vi "Downsample_Filter_Test.vi"() -> ()   [LabVIEW 2018]
uses:
  <vilib>/measure/maspectr.llb/Power Spectrum and PSD Export Mode.ctl
  <vilib>/measure/maspectr.llb/FFT Power Spectrum and PSD for 1 Chan.vi
  <vilib>/measure/NI_MAPro.lvlib
panel:
  out "original size":i32
  out "filtered size":i32
  out "Output valid":i16[](graph)
  out "filtered numeric":dbl[](array[numeric])
  out "Filtered signal":dbl[](graph)
  out "Power spectrum in":cluster{"f0":dbl, "df":dbl, "magnitude":dbl[]}(graph)
  out "Power spectrum out":cluster{"f0":dbl, "df":dbl, "magnitude":dbl[]}[](graph)
  out "Input signal":dbl[](graph)
  out "# of Iterations":i32
  out "# of samples":i32
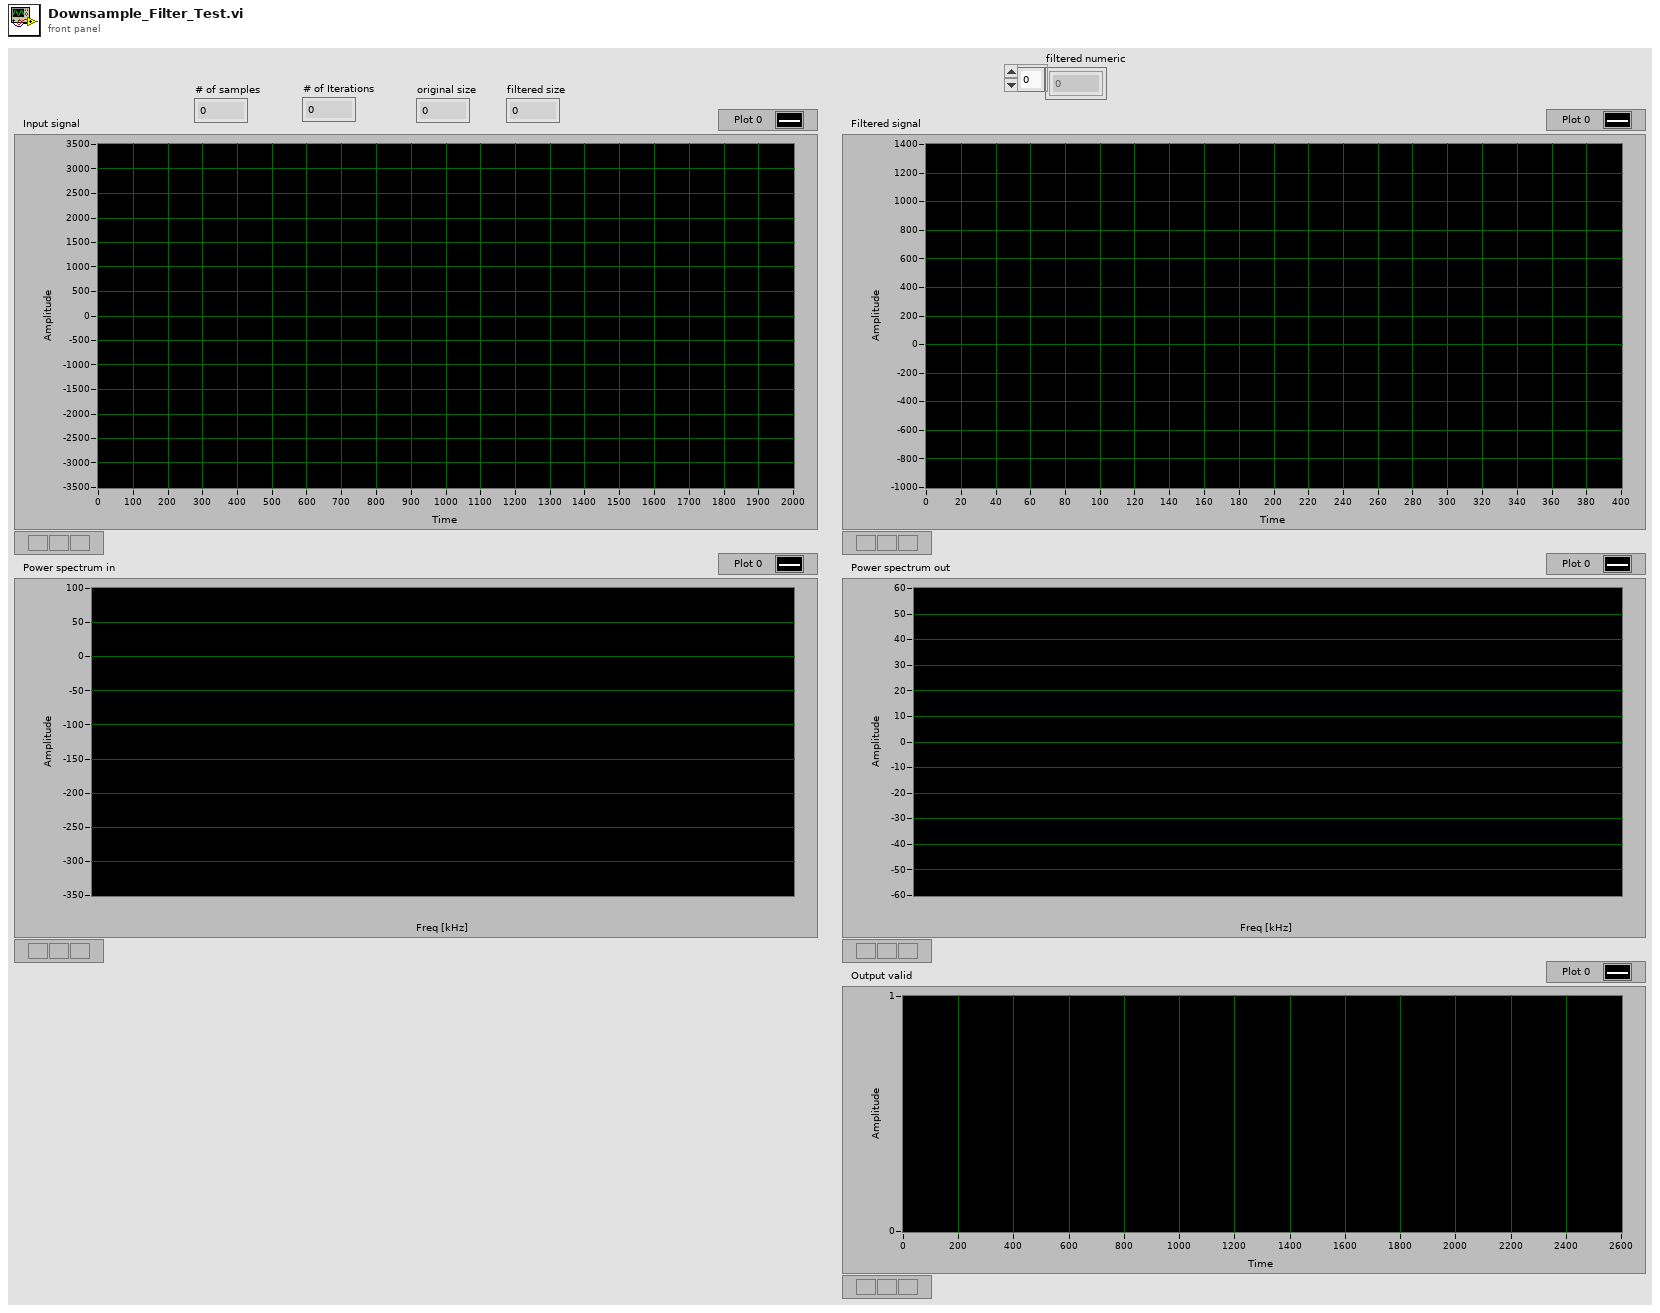
[diagram p1: front panel]
types:
  T1 = typedef "NI_MAPro.lvlib/Power Spectrum and PSD Export Mode.ctl" = u16
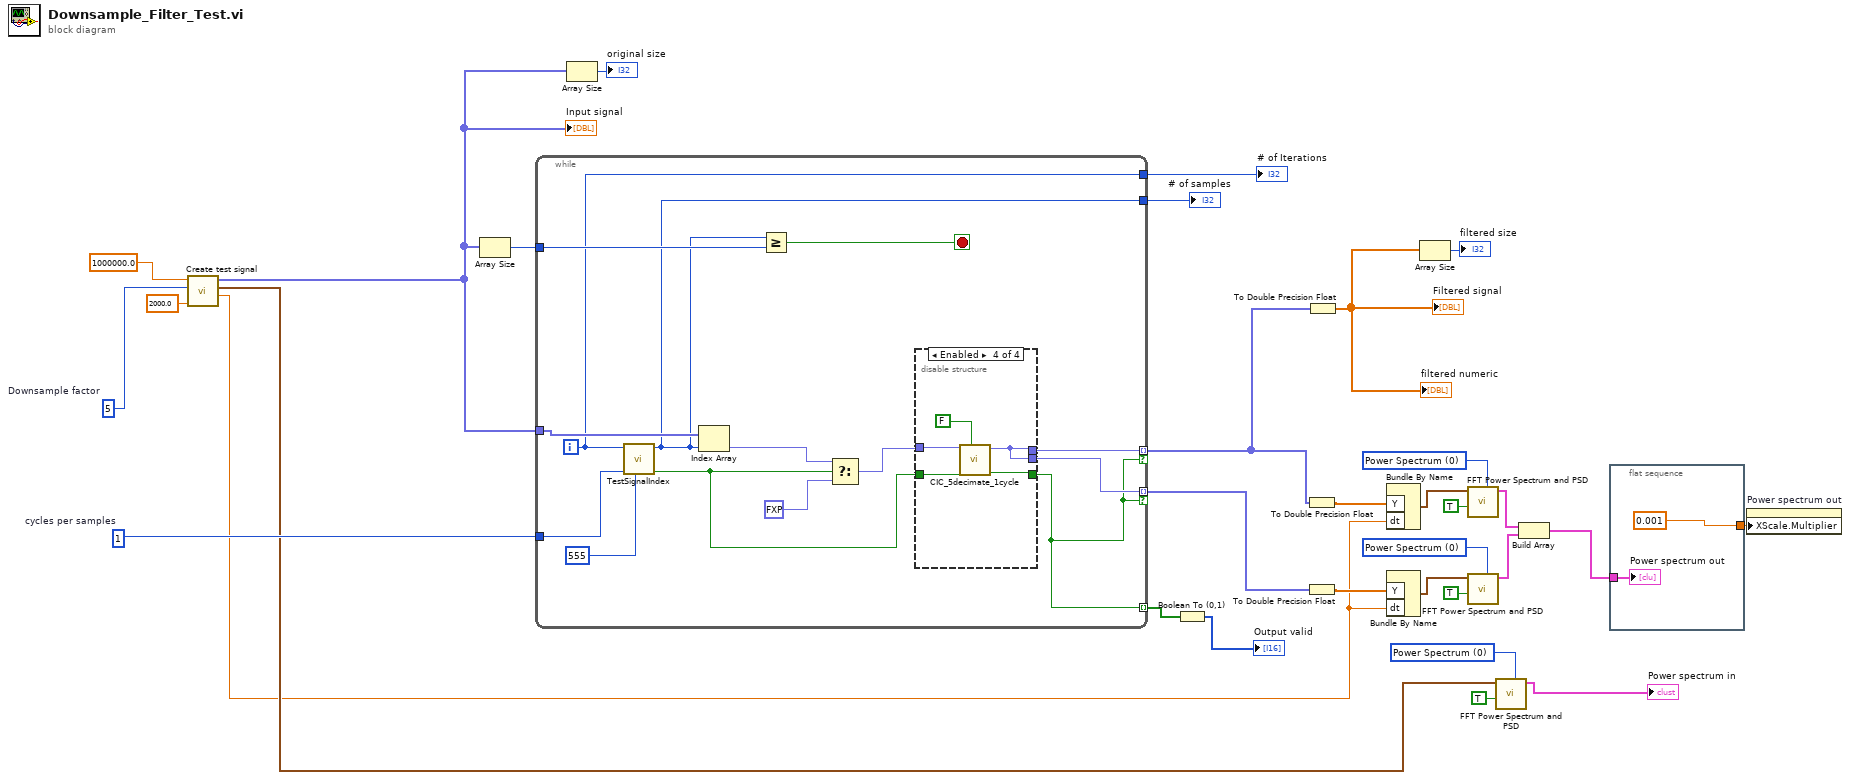
[diagram p0: block diagram]
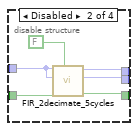
[diagram p3: hidden frame]
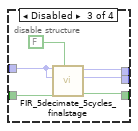
[diagram p4: hidden frame]
diagram:
  w15 = T1 0 items=["Power Spectrum", "Power Spectral Density"] ("export mode")
  w20 = 5  # Downsample factor
  w24 = 1  # cycles per samples
  w26 = T1 0 items=["Power Spectrum", "Power Spectral Density"] ("export mode")
  w30 = T1 0 items=["Power Spectrum", "Power Spectral Density"] ("export mode")
  n1 = call "Create test signal.vi"("Number of samples"=2000.0, "Downsample factor"=w20, "Sample rate"=1000000.0) -> ("dt"=w9:dbl, "signal out"=w22:waveform(dbl), "Y"=w4:fxp<+/-,16,14>[])  [unwired: 6 in]
  "Input signal" <- w4
  n2 = Array Size(array=w4) -> (size(s)=w32:i32)
  n3 = while {
    tunnel: w4 -> [w46]
    tunnel: [w43] -> w12 mode=indexing if=w35
    tunnel: w32 -> [w44]
    tunnel: w24 -> [w42]
    tunnel: [w35] -> w23 mode=indexing
    tunnel: [w36] -> w11 mode=indexing if=w35
    tunnel: [w34] -> w3
    tunnel: [w33] -> w2
    i -> [w33]
    stop <- w45 stop-if-true
    n4 = call "TestSignalIndex.vi"("initial delay"=555, "cycles per sample"=w42, "index"=w33) -> ("valid out"=w37:bool, "array index"=w34:i32)  [unwired: 7 in]
    n5 = Index Array(array=w46, index=w34) -> (element=w41:fxp<+/-,16,14>)
    n6 = Greater Or Equal?(x=w34, y=w44) -> (x >= y?=w45:bool)
    n7 = Select(t=w41, s=w37, f=fxp<+/-,16,14> 0.0) -> (s? t:f=w40:fxp<+/-,16,14>)
    n8 = disable-structure shown="Enabled" {
      disable-tunnel: [w51 w56 w62 w66] -> w43
      disable-tunnel: w40 -> [w50 w55 w61 w70]
      disable-tunnel: w37 -> [w49 w58 w64 w68]
      disable-tunnel: [w48 w54 w60 w66] -> w36
      disable-tunnel: [w47 w57 w63 w67] -> w35
      frame Disabled {
        n9 = flat-sequence {
          tunnel: [w53] -> w51
          tunnel: w50 -> [w53]
          tunnel: w49 -> [w52]
          tunnel: [w53] -> w48
          tunnel: [w52] -> w47
          frame #0 {
          }
        }
      }
      frame Disabled {
        n10 = call "FIR_2decimate_5cycles.vi"("reset"=FALSE, "valid in"=w58, "Q in"=w55, "I in"=w55) -> ("valid out"=w57:bool, "Q out"=w54:fxp<+/-,16,14>, "I out"=w56:fxp<+/-,16,14>)  [unwired: 4 in, 1 out]
      }
      frame Disabled {
        n11 = call "FIR_5decimate_5cycles_finalstage.vi"("reset"=FALSE, "valid in"=w64, "Q in"=w61, "I in"=w61) -> ("valid out"=w63:bool, "Q out"=w60:fxp<+/-,16,14>, "I out"=w62:fxp<+/-,16,14>)  [unwired: 4 in, 1 out]
      }
      frame Enabled {
        n12 = call "CIC_5decimate_1cycle.vi"("reset"=FALSE, "valid in"=w68, "Data in"=w70) -> ("valid out"=w67:bool, "Data out"=w66:fxp<+/-,16,14>)  [unwired: 7 in]
      }
    }
  }
  "# of samples" <- w3
  "# of Iterations" <- w2
  n13 = Array Size(array=w4) -> (size(s)=→"original size":i32)
  n14 = Boolean To (0,1)(Boolean=w23) -> (0, 1=→"Output valid":i16[])
  n15 = To Double Precision Float(number=w12) -> (double precision float=w18:dbl[])
  n16 = To Double Precision Float(number=w11) -> (double precision float=w28:dbl[])
  n17 = To Double Precision Float(number=w12) -> (double precision float=w7:dbl[])
  "Filtered signal" <- w7
  "filtered numeric" <- w7
  n18 = Bundle By Name("Y"=w18, "dt"=w9) -> (w16:waveform(dbl))  [unwired: 1 in]
  n19 = Bundle By Name("Y"=w28, "dt"=w9) -> (w31:waveform(dbl))  [unwired: 1 in]
  n20 = Array Size(array=w7) -> (size(s)=→"filtered size":i32)
  n21 = call-poly <vilib>:"FFT Power Spectrum and PSD.vi"("export mode"=w15, "dB On (F)"=TRUE, "time signal"=w16) -> ("Power Spectrum / PSD"=w13:cluster{"f0":dbl, "df":dbl, "magnitude":dbl[]})  [unwired: 5 in, 3 out]
  n22 = call-poly <vilib>:"FFT Power Spectrum and PSD.vi"("export mode"=w30, "dB On (F)"=TRUE, "time signal"=w31) -> ("Power Spectrum / PSD"=w14:cluster{"f0":dbl, "df":dbl, "magnitude":dbl[]})  [unwired: 5 in, 3 out]
  n23 = call-poly <vilib>:"FFT Power Spectrum and PSD.vi"("export mode"=w26, "dB On (F)"=TRUE, "time signal"=w22) -> ("Power Spectrum / PSD"=→"Power spectrum in":cluster{"f0":dbl, "df":dbl, "magnitude":dbl[]})  [unwired: 5 in, 3 out]
  n24 = Build Array(w13, w14) -> (w10:cluster{"f0":dbl, "df":dbl, "magnitude":dbl[]}[])
  n25 = flat-sequence {
    tunnel: w10 -> [w72]
    tunnel: [0.001 ("X Scale.Offset and Multiplier:Multiplier")] -> w8
    frame #0 {
      "Power spectrum out" <- w72
    }
  }
  n26 = property on="Power spectrum out" class="WFGraph (strict)"("XScale.Multiplier"=w8) -> ()  [unwired: 2 in, 2 out]
